vi "fit2.vi"(0 "array":dbl[][](array[numeric]), 5 "previous fit extern":dbl[](array[numeric])=[167.14051755898402, 39.154023858146694, 9.534043979855182, 46.30966986704069, 8.376343461684309, 10.31708372536886, 0.0], 11 "error in (no error)":errorcluster, 12 "disable fit":bool) -> (2 "number of function calls":i32, 3 "Fitting Time":u32, 4 "best nonlinear fit":dbl[](array[numeric]), 6 "best fit parameters":dbl[](array[numeric])=[167.14051755898402, 39.154023858146694, 9.534043979855182, 46.30966986704069, 8.376343461684309, 10.31708372536886, 0.0], 10 "residue":dbl, 14 "estimated parameters":dbl[](array[numeric]), 15 "error out":errorcluster)   [LabVIEW 2015]
uses:
  <vilib>/Analysis/6fits.llb/Curve Fitting Criteria.ctl
  <vilib>/Analysis/baseanly.llb/Real Determinant.vi
  <vilib>/Analysis/1siggen.llb/Ramp Pattern by Samples.vi
  <vilib>/gmath/NumericalOptimization/Nonlinear Curve Fit LM bound.vi
  <vilib>/gmath/NI_Gmath.lvlib
  <vilib>/Analysis/NI_AALPro.lvlib
  <vilib>/Analysis/NI_AALBase.lvlib
panel:
  in  "delta":dbl=2.0 format="%#_13g"
  out "Time (s)\nfI chart":u32(graph)
  out "Time (s)\nEstim. cycle Chart":dbl(graph)
  out "Time (s)\nEstim. cycle":dbl
  out "Estimation state":T1(ring)
  out "parameter cropped":T2={"parameter minimum"=[1.0, 0.0, 0.0, 1.0, 1.0, -720.0, 0.0], "parameter maximum"=[255.0, 640.0, 480.0, 80.0, 80.0, 720.0, 128.0]}
  in  "parameter initial":T2={"parameter minimum"=[1.0, 0.0, 0.0, 1.0, 1.0, -180.0, 0.0], "parameter maximum"=[255.0, 640.0, 480.0, 500.0, 500.0, 180.0, 128.0]}
  out "number of samples":T3
  in  "initial Alpha (DEG)":dbl=45.0
  in  "termination":cluster{"max iteration":i32, "tolerance":dbl}={"max iteration"=100, "tolerance"=1e-06}
  # "max Amplitude"
  # "Amplitude"
  # "x max"
  # "m1 (Mean 1)"
  # "y max"
  # "m2 (Mean 2)"
  # "Waist 1"
  # "wx Estimated"
  # "wy Estimated"
  # "Waist 2"
  # "alpha"
  # "PI (/2)"
  # "Offset"
  # "(0) Amplitude\n(1) X-Pos\n(2) Y-Pos\n(3) width A\n(4) Width B\n(5) angle (DEG)\n(6) Offset"
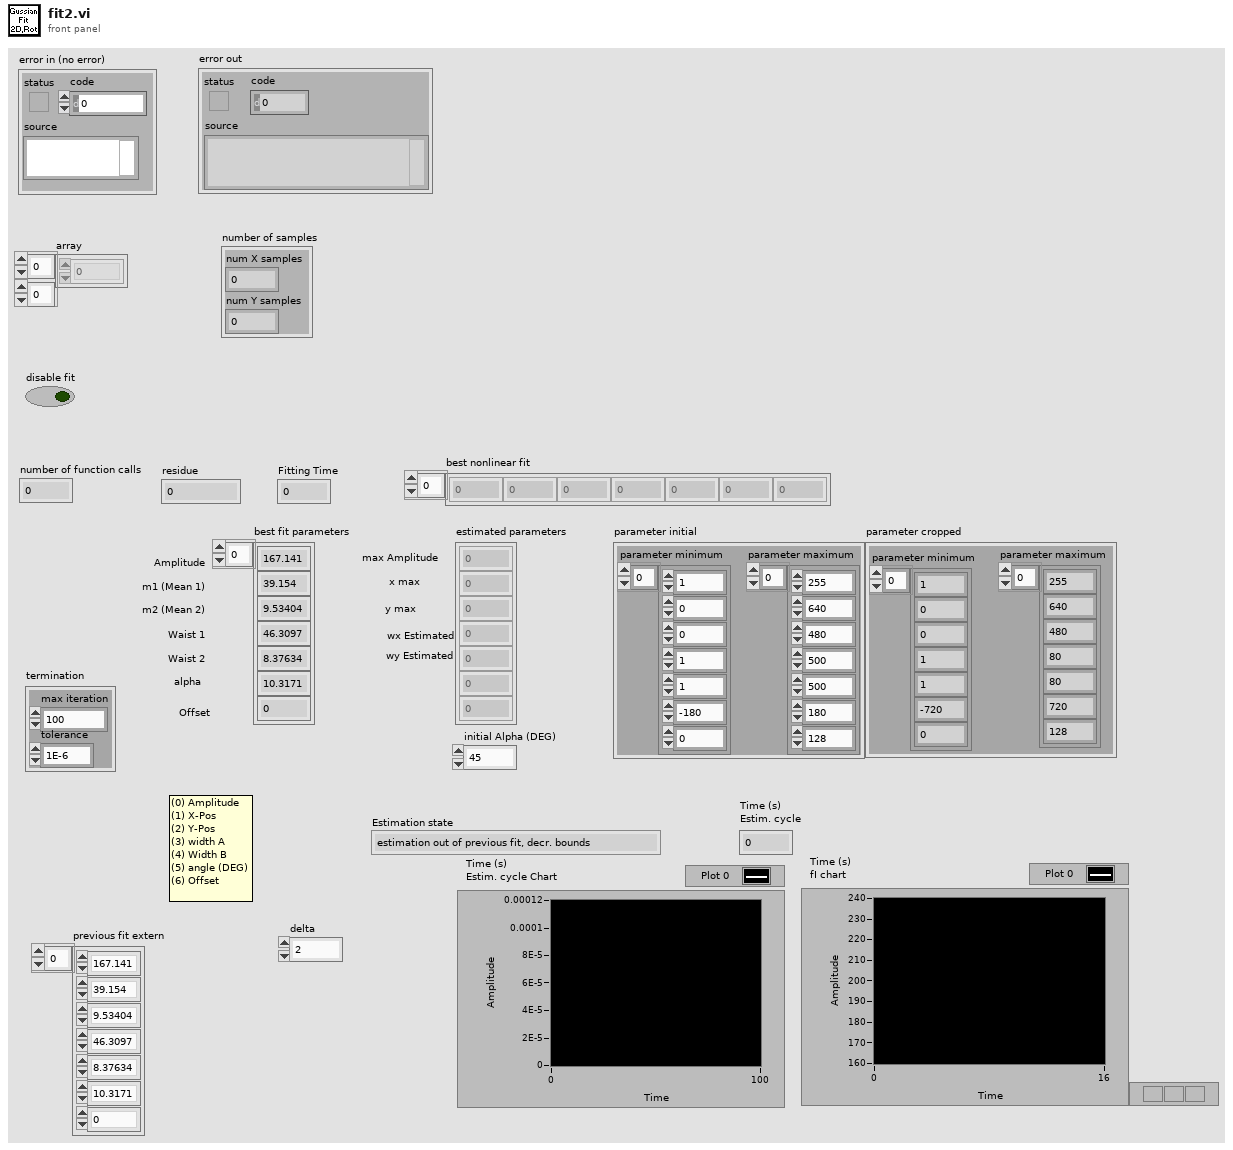
[diagram p1: front panel]
types:
  T1 = enum16{"estimation out of previous fit, decr. bounds", "estimation out of previous fit, same bounds", "New parameter estimation"}
  T2 = cluster{"parameter minimum":dbl[], "parameter maximum":dbl[]}
  T3 = cluster{"num X samples":i32, "num Y samples":i32}
  T4 = typedef "NI_AALPro.lvlib/Curve Fitting Criteria.ctl" = u16
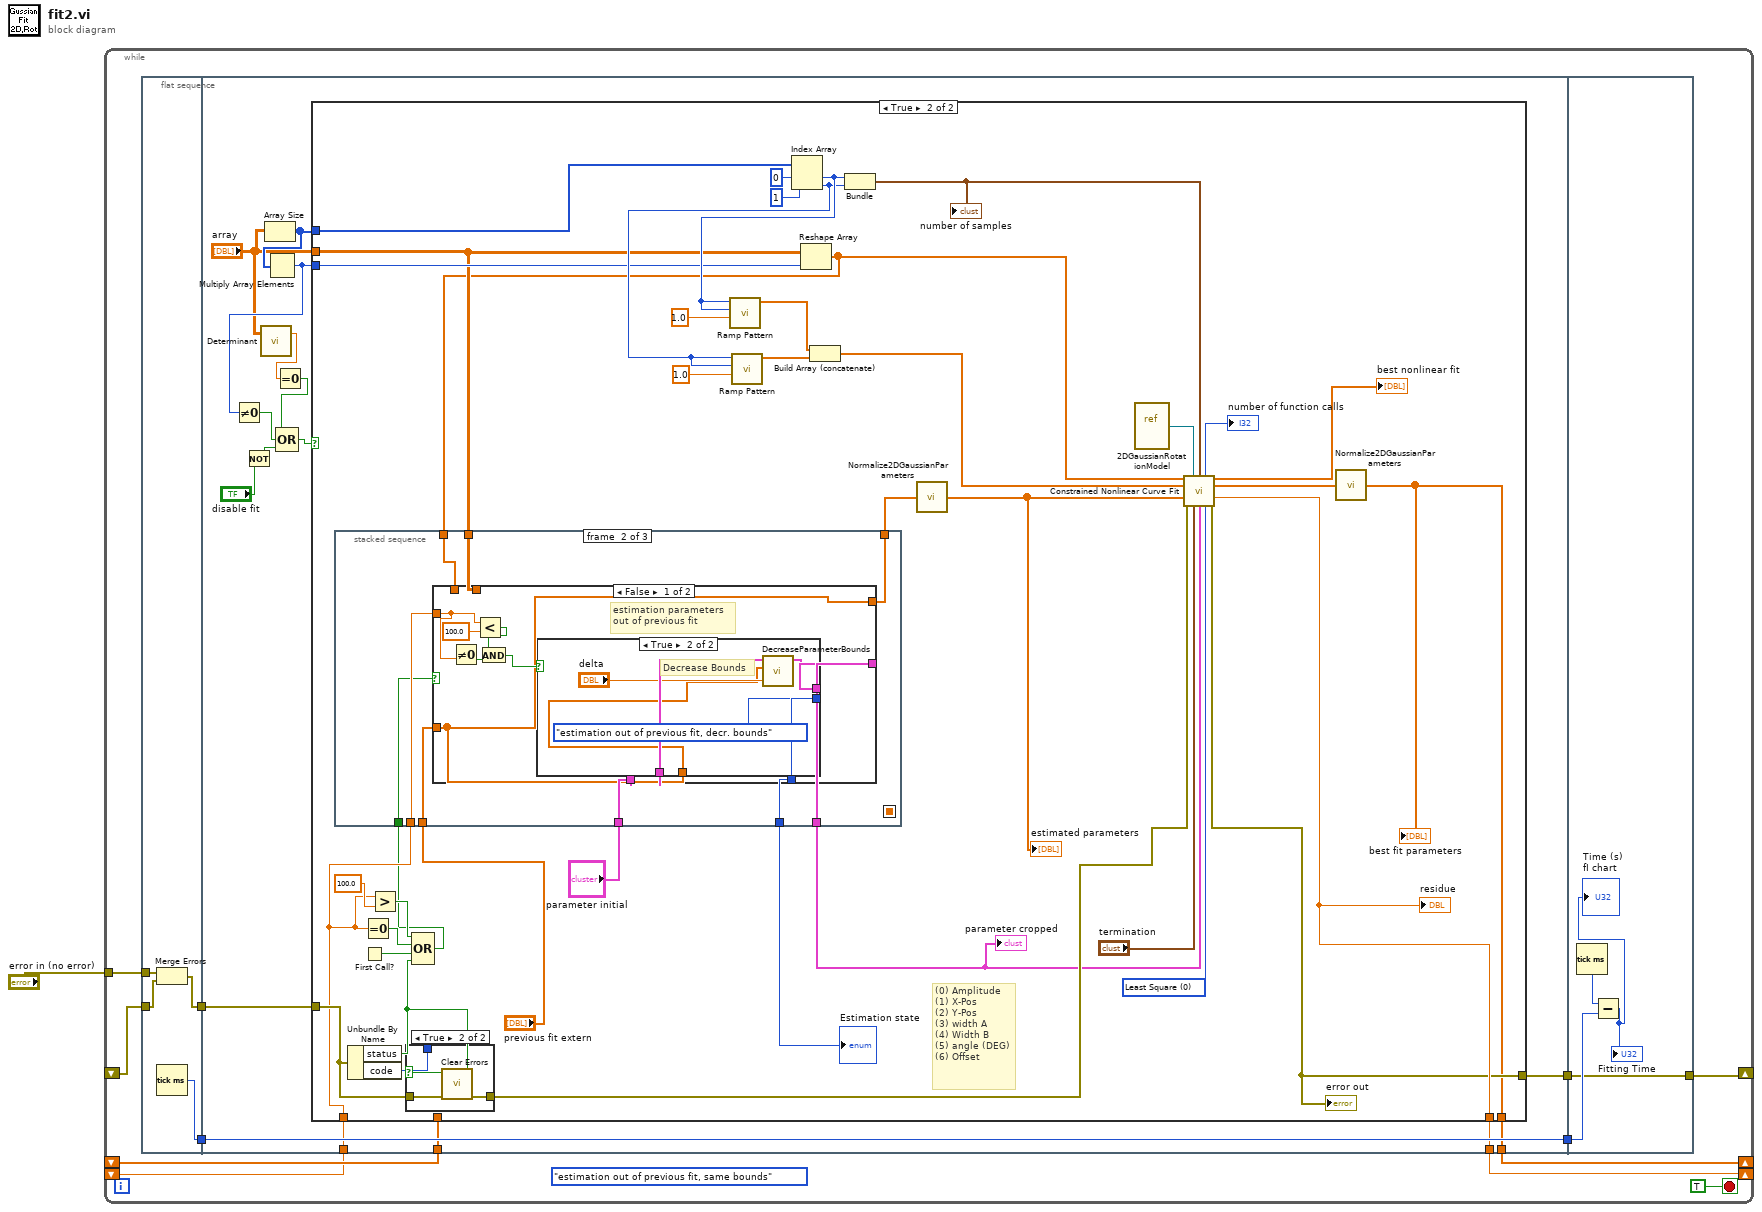
[diagram p0: block diagram]
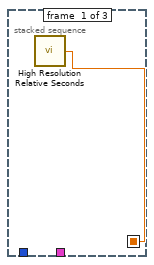
[diagram p3: hidden frame]
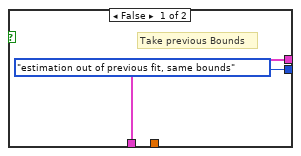
[diagram p4: hidden frame]
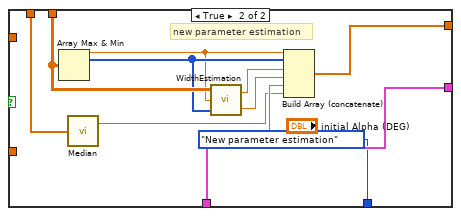
[diagram p5: hidden frame]
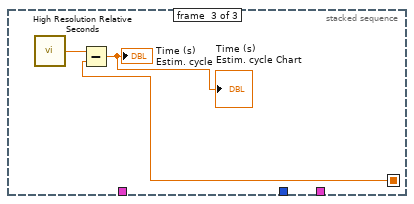
[diagram p6: hidden frame]
diagram:
  n1 = while {
    shift-right: [w10] -> _
    shift-left: _ -> [w9]
    shift-right: [w8] -> _
    shift-left: _ -> [w7]
    shift-right: [w6] -> _
    shift-left: _ -> [w4]
    tunnel: "error in (no error)" -> [w2]
    stop <- TRUE stop-if-true
    (unwired) T1."estimation out of previous fit, same bounds" ("Estimation state")
    n2 = flat-sequence {
      tunnel: [w17] -> w13
      tunnel: w4 -> [w16]
      tunnel: [w14] -> w3
      tunnel: w2 -> [w15]
      tunnel: w13 -> [w33]
      tunnel: [w33] -> w12
      tunnel: [w31] -> w10
      tunnel: w9 -> [w18]
      tunnel: [w32] -> w8
      tunnel: w7 -> [w28]
      tunnel: [w30] -> w5
      tunnel: w3 -> [w29]
      tunnel: w12 -> [w122]
      tunnel: [w121] -> w6
      tunnel: w5 -> [w121]
      frame #0 {
        n3 = Merge Errors(w15, w16) -> (w14:errorcluster)
        n4 = Tick Count (ms)() -> (millisecond timer value=w17:u32)
      }
      frame #1 {
        n5 = Not(x="disable fit") -> (.not. x?=w22:bool)
        n6 = call-poly <vilib>:"Determinant.vi"("Input Matrix"="array") -> ("determinant"=w20:dbl)  [unwired: 1 in, 1 out]
        n7 = Array Size(array="array") -> (size(s)=w24:i32[])
        n8 = Multiply Array Elements(1:w24) -> (0:w23:i32)
        n9 = Not Equal To 0?(x=w23) -> (x != 0?=w27:bool)
        n10 = Equal To 0?(x=w20) -> (x = 0?=w19:bool)
        n11 = Compound Arithmetic op=OR(w19, w27, w22) -> (w25:bool)
        n12 = case shown="True" w25 {
          tunnel: w24 -> [_ w66]
          tunnel: [w35 w61] -> w32
          tunnel: [w34 w47] -> w31
          tunnel: "array" -> [_ w46]
          tunnel: [w36 w56] -> w30
          tunnel: w29 -> [w36 w53]
          tunnel: w28 -> [w35 w44]
          tunnel: w23 -> [_ w51]
          tunnel: w18 -> [w34 _]
          frame False {
          }
          frame True {
            w68 = T4 0 items=["Least Square", "Least Absolute Residual", "Bisquare"] ("method")
            # "(0) Amplitude\n(1) X-Pos\n(2) Y-Pos\n(3) width A\n(4) Width B\n(5) angle (DEG)\n(6) Offset"
            n13 = Unbundle By Name(w53) -> ("status"=w55:bool, "code"=w54:i32)
            n14 = First Call?() -> (First Call?: T/F=w58:bool)
            n15 = Equal To 0?(x=w44) -> (x = 0?=w57:bool)
            n16 = Greater?(x=w44, y=100.0) -> (0:w59:bool)
            n17 = case shown="True" w55 {
              tunnel: w54 -> [_ w119]
              tunnel: w53 -> [w116 w118]
              tunnel: [w116 w117] -> w52
              frame False {
              }
              frame True {
                n18 = call <vilib>:"Clear Errors.vi"("error in (no error)"=w118, "specific error code to clear (0: all)"=w119) -> ("error out"=w117:errorcluster)  [unwired: 4 in, 1 out]
              }
            }
            n19 = Compound Arithmetic op=OR(w59, w57, w58, w55) -> (w43:bool)
            n20 = Index Array(array=w66, index #1=0 ("index"), index #2=1 ("index")) -> (element #1=w63:i32, element #2=w62:i32)
            n21 = call-poly <vilib>:"Ramp Pattern.vi"("start"=1.0, "end"=w63, "samples"=w63) -> ("Ramp Pattern"=w75:dbl[])  [unwired: 7 in, 1 out]
            n22 = call-poly <vilib>:"Ramp Pattern.vi"("start"=1.0, "end"=w62, "samples"=w62) -> ("Ramp Pattern"=w74:dbl[])  [unwired: 7 in, 1 out]
            n23 = Reshape Array(w46, w51) -> (w45:dbl[])
            n24 = stacked-sequence {
              seq-local: [w76 _ _] -> [_ _ w114]
              tunnel: w46 -> [_ w85 _]
              tunnel: w45 -> [_ w84 _]
              tunnel: w44 -> [_ w83 _]
              tunnel: w43 -> [_ w77 _]
              tunnel: "previous fit extern" -> [_ w82 _]
              tunnel: "parameter initial" -> [_ w81 _]
              tunnel: [_ w80 _] -> w41
              tunnel: [_ w79 _] -> w40
              tunnel: [_ w78 _] -> w39
              frame #0 {
                n25 = call <vilib>:"High Resolution Relative Seconds.vi"() -> ("relative seconds"=w76:dbl)
              }
              frame #1 {
                n26 = case shown="False" w77 {
                  tunnel: [w86 w106] -> w79
                  tunnel: w85 -> [_ w111]
                  tunnel: w82 -> [w86 _]
                  tunnel: w84 -> [_ w105]
                  tunnel: w83 -> [w93 _]
                  tunnel: [w90 w103] -> w78
                  tunnel: w81 -> [w89 w103]
                  tunnel: [w88 T1."New parameter estimation" ("Estimation state")] -> w80
                  frame False {
                    # "estimation parameters \nout of previous fit"
                    n27 = Not Equal To 0?(x=w93) -> (x != 0?=w92:bool)
                    n28 = Less?(x=w93, y=100.0) -> (x < y?=w91:bool)
                    n29 = And(x=w91, y=w92) -> (x .and. y?=w87:bool)
                    n30 = case shown="True" w87 {
                      tunnel: w89 -> [w96 w101]
                      tunnel: [w96 w100] -> w90
                      tunnel: w86 -> [_ w97]
                      tunnel: [T1."estimation out of previous fit, same bounds" ("Estimation state") T1."estimation out of previous fit, decr. bounds" ("Estimation state")] -> w88
                      frame False {
                        # "Take previous Bounds"
                      }
                      frame True {
                        # "Decrease Bounds"
                        n31 = call "DecreaseParameterBounds.vi"("delta"="delta", "Best Fits"=w97, "parameter bounds in"=w101) -> ("parameter bounds out"=w100:T2)  [unwired: 8 in]
                      }
                    }
                  }
                  frame True {
                    # "new parameter estimation"
                    n32 = Array Max & Min(array=w111) -> (max value=w107:dbl, max index (indices)=w110:i32[])  [unwired: 2 out]
                    n33 = call <vilib>:"Median.vi"("X"=w105) -> ("median"=w104:dbl)  [unwired: 1 out]
                    n34 = call "WidthEstimation.vi"("maximum index"=w110, "maximium"=w107, "2D Gaussian Data"=w111) -> ("wy Estimated"=w108:dbl, "wx Estimated"=w109:dbl)
                    n35 = Build Array (concatenate)(w107, w110, w109, w108, "initial Alpha (DEG)", w104) -> (w106:dbl[])
                  }
                }
              }
              frame #2 {
                n36 = call <vilib>:"High Resolution Relative Seconds.vi"() -> ("relative seconds"=w115:dbl)
                n37 = Subtract(x=w115, y=w114) -> (x-y=→"Time (s)\nEstim. cycle" →"Time (s)\nEstim. cycle Chart":dbl)
              }
            }
            "parameter cropped" <- w39
            "Estimation state" <- w41
            n38 = Build Array (concatenate)(w75, w74) -> (w69:dbl[])
            n39 = Bundle(w63, w62) -> (w67:cluster{i32, i32})  [unwired: 1 out]
            "number of samples" <- w67
            n40 = call "Normalize2DGaussianParameters.vi"("best fit parameters IN"=w40) -> ("best fit parameters OUT"=w50:dbl[])
            "estimated parameters" <- w50
            n41 = vi-ref "2DGaussianRotationModel.vi"() -> (w37:refnum<vi>)
            n42 = call-poly <vilib>:"Constrained Nonlinear Curve Fit.vi"("Y"=w45, "f(x,a)"=w37, "data"=w67, "X"=w69, "initial parameters"=w50, "error in (no error)"=w52, "termination"="termination", "parameter bounds"=w39, "method"=w68) -> ("number of function calls"=→"number of function calls":i32, "best nonlinear fit"=→"best nonlinear fit":dbl[], "best fit parameters"=w48:dbl[], "residue"=w61:dbl, "error out"=w56:errorcluster)  [unwired: 1 in, 1 out]
            "error out" <- w56
            "residue" <- w61
            n43 = call "Normalize2DGaussianParameters.vi"("best fit parameters IN"=w48) -> ("best fit parameters OUT"=w47:dbl[])
            "best fit parameters" <- w47
          }
        }
      }
      frame #2 {
        n44 = Tick Count (ms)() -> (millisecond timer value=w123:u32)
        n45 = Subtract(x=w123, y=w122) -> (x-y=→"Fitting Time" →"Time (s)\nfI chart":u32)
      }
    }
  }
